vi "Focus Index.vi"(5 "Pre-bin 2":bool=TRUE, 7 "Limit area":bool=TRUE, 8 "Smoothing radius 2":u16=2, 9 "Smoothing radius 1":u16=1, 11 "Input":dbl[][](graph)) -> (0 "Eval area":dbl[][](graph), 3 "Focus index":sgl format="%#_6f")   [LabVIEW 2018]
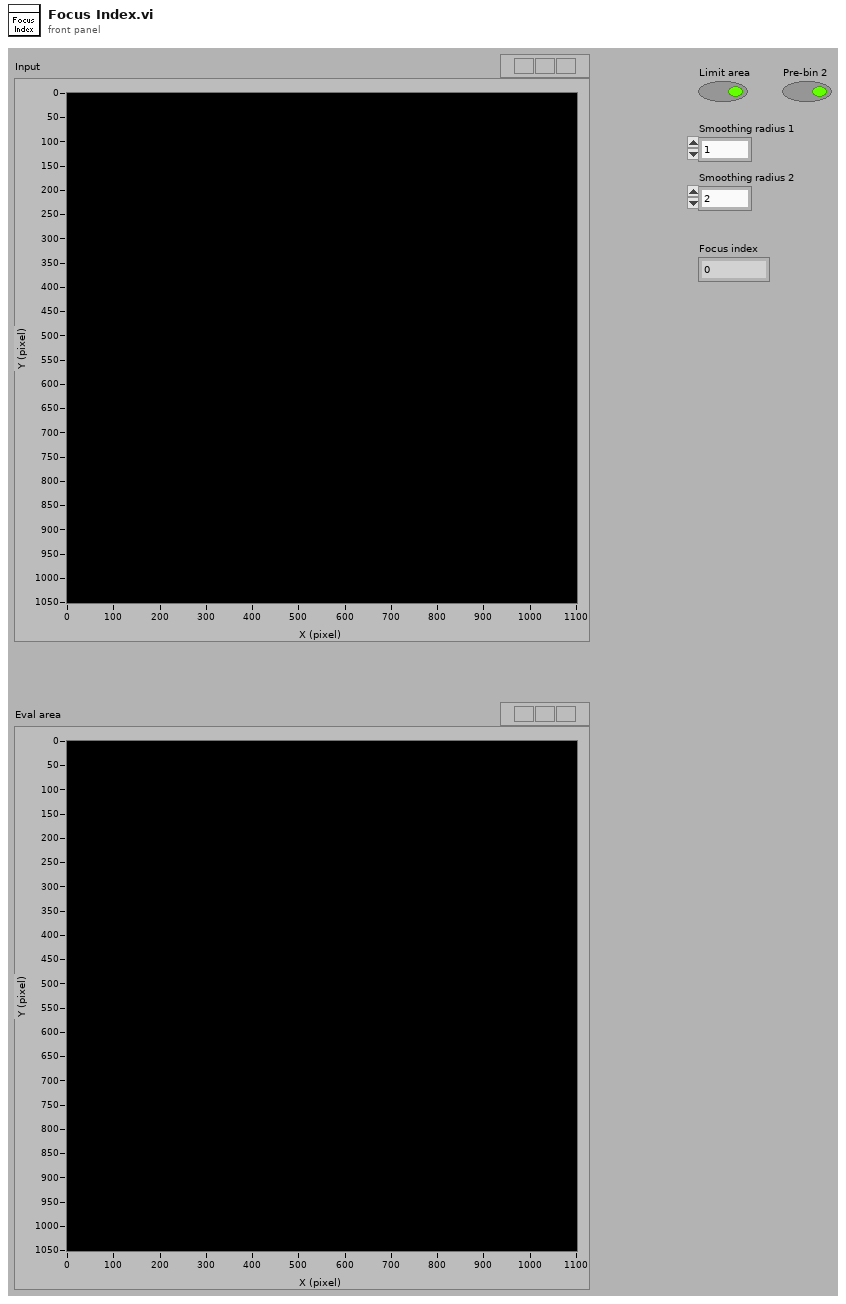
[diagram p1: front panel]
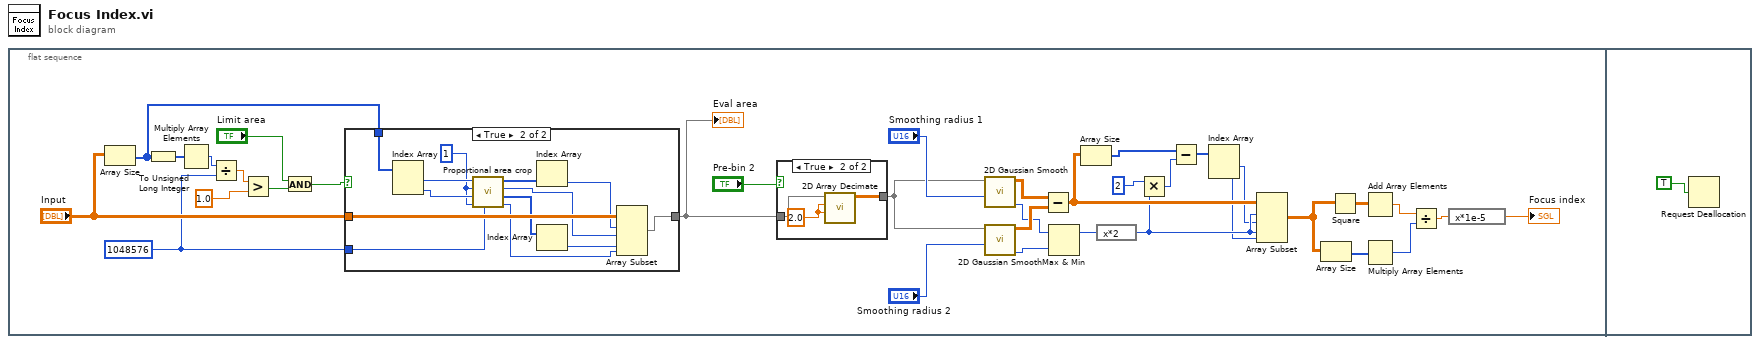
[diagram p0: block diagram]
diagram:
  n1 = flat-sequence {
    frame #0 {
      w5 = u32 1048576 ("y")
      n2 = Array Size(array="Input") -> (size(s)=w4:i32[])
      n3 = To Unsigned Long Integer(number=w4) -> (unsigned 32bit integer=w6:u32[])
      n4 = Multiply Array Elements(1:w6) -> (0:w21:u32)
      n5 = Divide(x=w21, y=w5) -> (x/y=w15:dbl)
      n6 = Greater?(x=w15, y=1.0) -> (0:w17:bool)
      n7 = And(x="Limit area", y=w17) -> (x .and. y?=w20:bool)
      n8 = case shown="True" w20 {
        tunnel: [w40 w52] -> w2
        tunnel: "Input" -> [w40 w53]
        tunnel: w5 -> [_ w47]
        tunnel: w4 -> [_ w46]
        frame False {
        }
        frame True {
          w45 = u8 1 ("X grids")
          n9 = Index Array(array=w46) -> (element #1=w51:i32, element #2=w50:i32)  [unwired: 2 in]
          n10 = call "Proportional area crop.vi"("Cropped to area pixels"=w47, "Y grids"=w45, "Y resolution"=w50, "X grids"=w45, "X resolution"=w51) -> ("Y length"=w48:u32, "Y index"=w41:u32[], "X length"=w49:u32, "X index"=w44:u32[])  [unwired: 3 in]
          n11 = Index Array(array=w44) -> (element=w43:u32)  [unwired: 1 in]
          n12 = Index Array(array=w41) -> (element=w42:u32)  [unwired: 1 in]
          n13 = Array Subset(array=w53, index (row)=w43, length (row)=w49, index (col)=w42, length (col)=w48) -> (w52:dbl[][])
        }
      }
      "Eval area" <- w2
      n14 = case shown="True" "Pre-bin 2" {
        tunnel: w2 -> [w36 w38]
        tunnel: [w36 w37] -> w1
        frame False {
        }
        frame True {
          w39 = 2.0 ("x decimating factor")
          n15 = call "2D Array Decimate.vi"("y decimating factor"=w39, "x decimating factor"=w39, "Input 2D Array"=w38) -> ("output array"=w37:dbl[][])  [unwired: 6 in, 2 out]
        }
      }
      n16 = call "2D Gaussian Smooth.vi"("radius"="Smoothing radius 1", "Input"=w1) -> ("Margin"=w25:u16, "Output"=w33:dbl[][])  [unwired: 8 in]
      n17 = call "2D Gaussian Smooth.vi"("radius"="Smoothing radius 2", "Input"=w1) -> ("Margin"=w24:u16, "Output"=w30:dbl[][])  [unwired: 8 in]
      n18 = Subtract(x=w33, y=w30) -> (x-y=w14:dbl[][])
      n19 = Max & Min(x=w25, y=w24) -> (max(x,y)=w23:u16)  [unwired: 1 out]
      n20 = Array Size(array=w14) -> (size(s)=w13:i32[])
      n21 = expression code="x*2"(w23) -> (w12:u16)
      n22 = Multiply(x=u16 2, y=w12) -> (x*y=w10:u16)
      n23 = Subtract(x=w13, y=w10) -> (x-y=w9:i32[])
      n24 = Index Array(array=w9) -> (element #1=w8:i32, element #2=w7:i32)  [unwired: 2 in]
      n25 = Array Subset(array=w14, index (row)=w12, length (row)=w8, index (col)=w12, length (col)=w7) -> (w26:dbl[][])
      n26 = Array Size(array=w26) -> (size(s)=w29:i32[])
      n27 = Square(x=w26) -> (x^2=w32:dbl[][])
      n28 = Add Array Elements(numeric array=w32) -> (sum=w31:dbl)
      n29 = Multiply Array Elements(1:w29) -> (0:w28:i32)
      n30 = Divide(x=w31, y=w28) -> (x/y=w27:dbl)
      n31 = expression code="x*1e-5"(w27) -> (→"Focus index":dbl)
    }
    frame #1 {
      n32 = Request Deallocation(TRUE ("flag")) -> ()
    }
  }
